vi "Image.vi"(2 "XRef":refnum<vi>, 3 "State In":T1) -> (0 "Image":picture)   [LabVIEW 2012, in "OpenG Remove Duplicates from 1 D Array.xnode"]
uses:
  OpenG Remove Duplicates from 1 D Array.xnode
  State.ctl
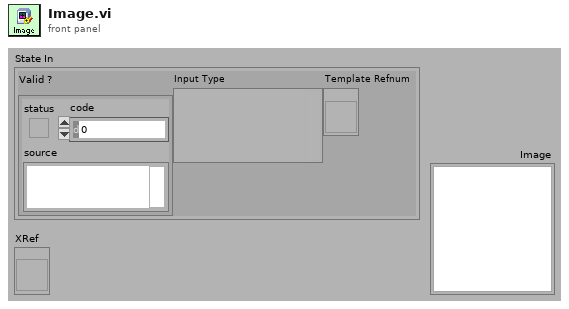
[diagram p1: front panel]
types:
  T1 = typedef "OpenG Remove Duplicates from 1 D Array.xnode/State.ctl" = cluster{"Valid ?":errorcluster, "Input Type":variant, "Template Refnum":refnum<vi>}
  T2 = typedef "imagedata.ctl" = cluster{"image type":i32, "image depth":i32, "image":u8[], "mask":u8[], "colors":u32[], "Rectangle":cluster{"left":i16, "top":i16, "right":i16, "bottom":i16}}
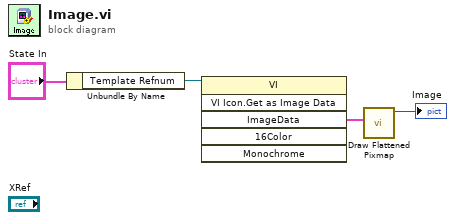
[diagram p0: block diagram]
diagram:
  n1 = Unbundle By Name("State In") -> ("Template Refnum"=w2:refnum<vi>)
  n2 = invoke class="VI" method="VI Icon.Get as Image Data"(reference=w2) -> ("ImageData"=w1:T2)  [unwired: 5 in, 5 out]
  n3 = call <vilib>:"Draw Flattened Pixmap.vi"("image data"=w1) -> ("new picture"=→"Image":picture)  [unwired: 1 in, 7 out]
